vi "Close.vi"(8 "error in (no error)":errorcluster, 11 "Communication in":refnum<class "Communication.lvclass">) -> (0 "error out":errorcluster, 3 "Communication out":refnum<class "Communication.lvclass">)   [LabVIEW 2019, in "Communication.lvclass"]
uses:
  Communication.lvclass
  Communication.lvclass/Communication.ctl
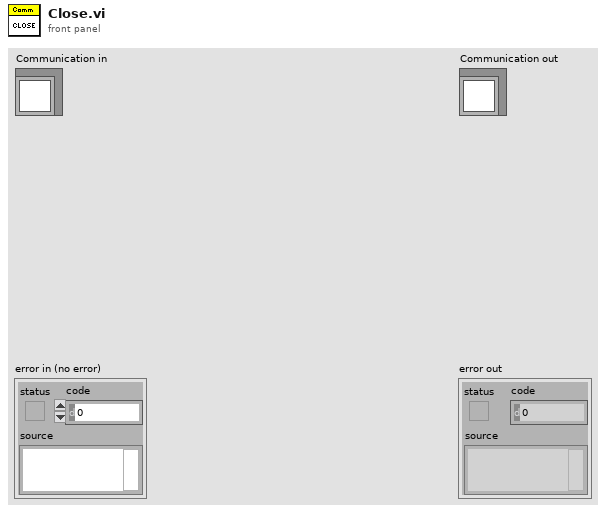
[diagram p1: front panel]
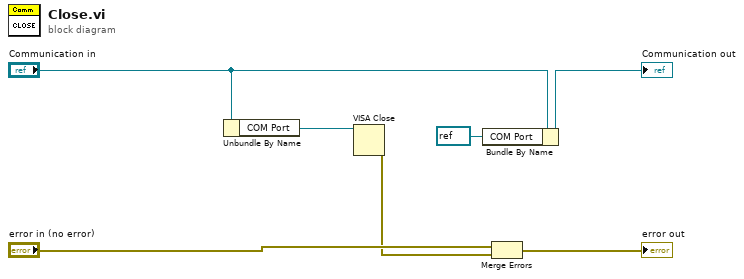
[diagram p0: block diagram]
diagram:
  n1 = Unbundle By Name("Communication in") -> ("COM Port"=w5:refnum<visa-resource-name>)
  n2 = VISA Close(VISA resource name=w5) -> (error out=w2:errorcluster)  [unwired: 1 in]
  n3 = Bundle By Name(cluster="Communication in", "COM Port"=refnum<visa-resource-name> refnum) -> (→"Communication out":refnum<class "Communication.lvclass">)
  n4 = Merge Errors("error in (no error)", w2) -> (→"error out":errorcluster)
